vi "Add Sub Build Spec.vi"(0 "NI Build Specification in":refnum<class "NI Build Specification_LV.lvclass">, 5 "Sub Buiild Specification":refnum<class "NI Build Specification_LV.lvclass">, 11 "error in (no error)":errorcluster) -> (4 "NI Build Specification out":refnum<class "NI Build Specification_LV.lvclass">, 15 "error out":errorcluster)   [LabVIEW 2017, in "CL_G3_VIComponentBuilder.lvlib" / "NI Build Specification_LV.lvclass"]
doc: "Adds a sub build spec to the <Anchor><Text>Sub Build Specs</Text><AnchorName>Sub Build Specs</AnchorName><PageName>NI Build Specification_LV Class Documentation</PageName><Space>TCS</Space></Anchor> lookup table."
uses:
  NI Build Specification_LV.lvclass
  NI Build Specification_LV.lvclass/NI Build Specification_LV.ctl
  Accessors/Read Export's Build Spec Name.vi
  Accessors/Read Sub Build Specs.vi
  Accessors/Write Sub Build Specs.vi
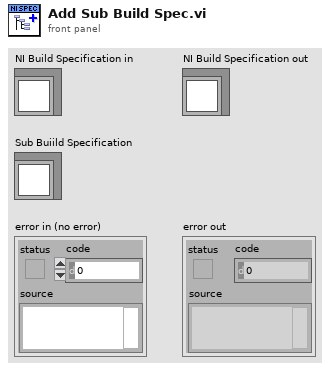
[diagram p1: front panel]
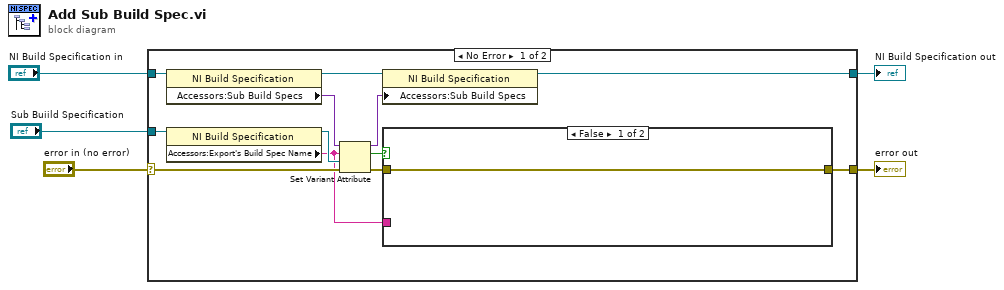
[diagram p0: block diagram]
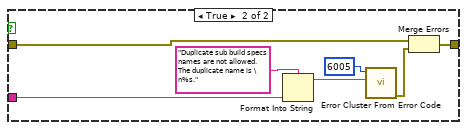
[diagram p2: hidden frame]
diagram:
  n1 = case shown="No Error" "error in (no error)" {
    selector: "error in (no error)" -> [w8 w27]
    tunnel: [w6 w27] -> w4
    tunnel: [w12 w26] -> w2
    tunnel: "NI Build Specification in" -> [w17 w26]
    tunnel: "Sub Buiild Specification" -> [w14 _]
    frame No Error {
      n2 = property class="NI Build Specification"(reference=w17) -> (reference out=w16:refnum<class "NI Build Specification_LV.lvclass">, "Accessors:Sub Build Specs"=w15:variant)  [unwired: 1 in, 1 out]
      n3 = property class="NI Build Specification"(reference=w14) -> (reference out=w13:refnum<class "NI Build Specification_LV.lvclass">, "Accessors:Export's Build Spec Name"=w7:string)  [unwired: 1 in, 1 out]
      n4 = Set Variant Attribute(Variant=w15, name=w7, value=w13, error in=w8) -> (Variant out=w11:variant, replaced=w10:bool, error out=w9:errorcluster)
      n5 = property class="NI Build Specification"(reference=w16, "Accessors:Sub Build Specs"=w11) -> (reference out=w12:refnum<class "NI Build Specification_LV.lvclass">)  [unwired: 1 in, 1 out]
      n6 = case shown="False" w10 {
        tunnel: w9 -> [w18 w25]
        tunnel: w7 -> [_ w22]
        tunnel: [w18 w19] -> w6
        frame False {
        }
        frame True {
          n7 = Format Into String(format string="Duplicate sub build specs names are not allowed. The duplicate name is \n%s.", w22) -> (resulting string=w21:string)  [unwired: 2 in, 1 out]
          n8 = call <vilib>:"Error Cluster From Error Code.vi"("error message (\"\")"=w21, "error code (0)"=6005) -> ("error out"=w24:errorcluster)  [unwired: 7 in]
          n9 = Merge Errors(w25, w24) -> (w19:errorcluster)
        }
      }
    }
    frame Error {
    }
  }
  "error out" <- w4
  "NI Build Specification out" <- w2
